vi "GetLUTModeList.vi"(10 "List":u32) -> (2 "GetLUTModeList":cluster{string, i32})   [LabVIEW 2015]
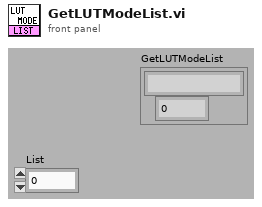
[diagram p1: front panel]
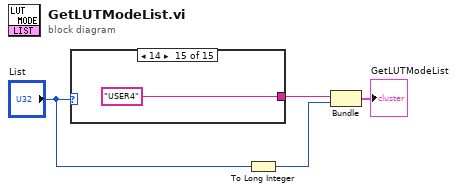
[diagram p0: block diagram]
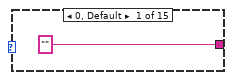
[diagram p2: hidden frame]
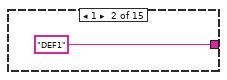
[diagram p3: hidden frame]
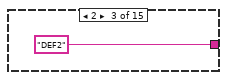
[diagram p4: hidden frame]
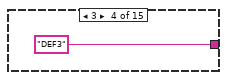
[diagram p5: hidden frame]
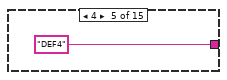
[diagram p6: hidden frame]
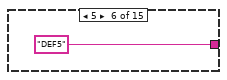
[diagram p7: hidden frame]
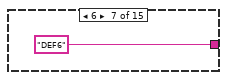
[diagram p8: hidden frame]
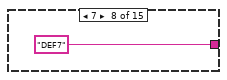
[diagram p9: hidden frame]
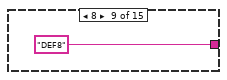
[diagram p10: hidden frame]
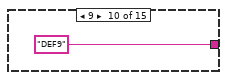
[diagram p11: hidden frame]
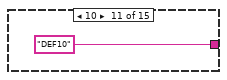
[diagram p12: hidden frame]
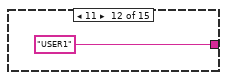
[diagram p13: hidden frame]
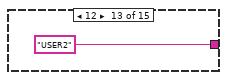
[diagram p14: hidden frame]
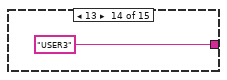
[diagram p15: hidden frame]
diagram:
  n1 = case shown="14" "List" {
    tunnel: ["" "DEF1" "DEF2" "DEF3" "DEF4" "DEF5" "DEF6" "DEF7" "DEF8" "DEF9" "DEF10" "USER1" "USER2" "USER3" "USER4"] -> w3
    frame 0, Default {
    }
    frame 1 {
    }
    frame 2 {
    }
    frame 3 {
    }
    frame 4 {
    }
    frame 5 {
    }
    frame 6 {
    }
    frame 7 {
    }
    frame 8 {
    }
    frame 9 {
    }
    frame 10 {
    }
    frame 11 {
    }
    frame 12 {
    }
    frame 13 {
    }
    frame 14 {
    }
  }
  n2 = To Long Integer(number="List") -> (32bit integer=w2:i32)
  n3 = Bundle(w3, w2) -> (→"GetLUTModeList":cluster{string, i32})  [unwired: 1 out]
